vi "close all.vi"(8 "error in (no error)":errorcluster, 11 "5785_2_x_200MHz in":refnum<class "5785_2_x_200MHz.lvclass">) -> (0 "error out":errorcluster, 3 "5785_2_x_200MHz out":refnum<class "5785_2_x_200MHz.lvclass">)   [LabVIEW 2021, in "5785_2_x_200MHz.lvclass"]
uses:
  5785_2_x_200MHz.lvclass
  5785_2_x_200MHz.lvclass/5785_2_x_200MHz.ctl
  <vilib>/rvi/interface/nirviCloseFPGA/nirviCloseFPGA.xnode
  <vilib>/FPGAPlugInAG/Dynamic/niLvFpga_Close_Dynamic.vi
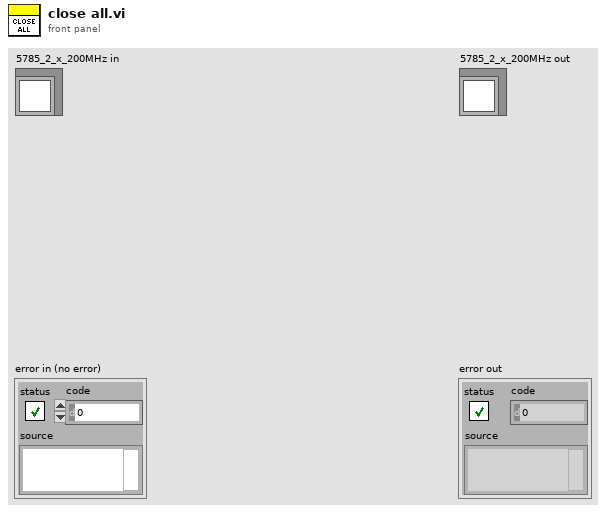
[diagram p1: front panel]
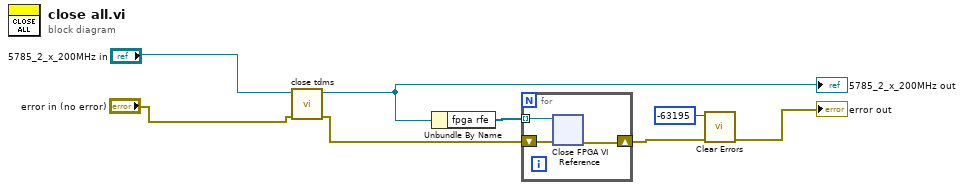
[diagram p0: block diagram]
diagram:
  n1 = call-dynamic "close tdms.vi"("error in (no error)"="error in (no error)", "device_type in"="5785_2_x_200MHz in") -> ("error out"=w2:errorcluster, "device_type out"=w1:refnum<class "5785_2_x_200MHz.lvclass">)  [unwired: 8 in]
  "5785_2_x_200MHz out" <- w1
  n2 = Unbundle By Name(w1) -> ("fpga rfe"=w8:refnum<k20>[])
  n3 = for {
    shift-right: [w10] -> w6
    shift-left: w2 -> [w11]
    tunnel: w8 -> [w9] mode=indexing
    n4 = xnode "Close FPGA VI Reference"("FPGA VI Reference In"=w9, "error in"=w11) -> ("error out"=w10:errorcluster)
  }
  n5 = call <vilib>:"Clear Errors.vi"("error in (no error)"=w6, "specific error code to clear (0: all)"=-63195) -> ("error out"=→"error out":errorcluster)  [unwired: 4 in, 1 out]
